vi "Write CAN Frame.vi"(8 "error in (no error)":errorcluster, 10 "data":T1[](array[typedef]) {"payload" format="%x"; "timestamp" format="%<%.7X\n%x>T"; "type" items=["CAN Data"=0, "CAN Remote"=1, "CAN Bus Error"=2, "CAN 2.0 Data"=8, "CAN FD Data"=16, "CAN FD+BRS Data"=24, "J1939 Data"=192, "Delay"=224, "Log Trigger"=225, "Start Trigger"=226]; "identifier" format="%x"}, 11 "PXI 8513 in":refnum<class "PXI 8513.lvclass">) -> (0 "error out":errorcluster, 3 "PXI 8513 out":refnum<class "PXI 8513.lvclass">)   [LabVIEW 2016, in "CAN.lvlib" / "PXI 8513.lvclass"]
uses:
  PXI 8513.lvclass
  <vilib>/xnet/xnet.llb/XNET Frame CAN.ctl
  <vilib>/xnet/xnet.llb/XNET Frame Type CAN.ctl
  PXI 8513.lvclass/PXI 8513.ctl
  <vilib>/xnet/xnet.llb/XNET Write (Frame CAN).vi
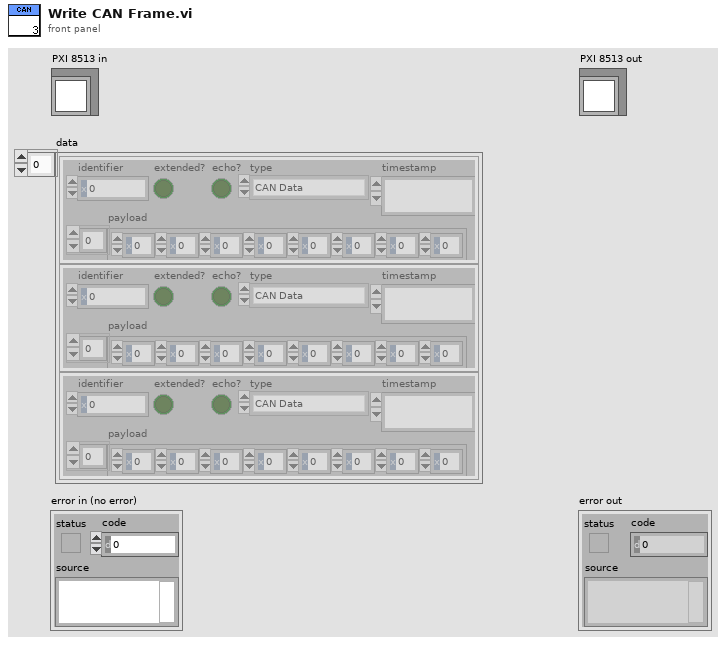
[diagram p1: front panel]
types:
  T1 = typedef "XNET Frame CAN.ctl" = cluster{"timestamp":timestamp, "payload":u8[], "identifier":u32, "type":T2, "extended?":bool, "echo?":bool}
  T2 = typedef "XNET Frame Type CAN.ctl" = u8
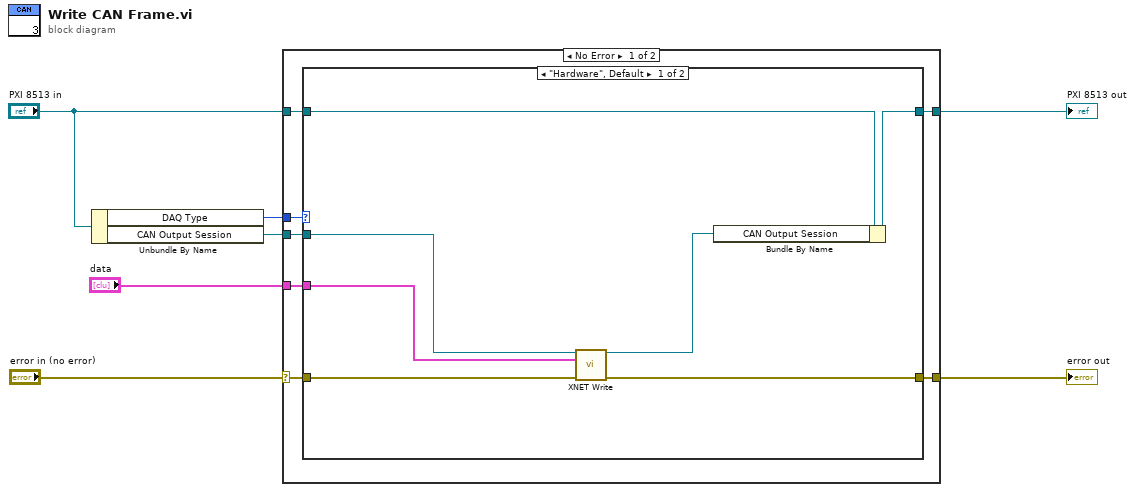
[diagram p0: block diagram]
diagram:
  n1 = Unbundle By Name("PXI 8513 in") -> ("DAQ Type"=w5:enum16{"Hardware", "Simulation"}, "CAN Output Session"=w4:refnum<k21>)
  n2 = case shown="No Error" "error in (no error)" {
    selector: "error in (no error)" -> [w13 w24]
    tunnel: "PXI 8513 in" -> [w10 w25]
    tunnel: w5 -> [w14 _]
    tunnel: w4 -> [w12 _]
    tunnel: "data" -> [w11 _]
    tunnel: [w9 w25] -> w2
    tunnel: [w8 w24] -> w1
    frame No Error {
      n3 = case shown="\"Hardware\", Default" w14 {
        tunnel: w13 -> [w21 w22]
        tunnel: w12 -> [w20 _]
        tunnel: w11 -> [w19 _]
        tunnel: w10 -> [w18 w23]
        tunnel: [w16 w23] -> w9
        tunnel: [w17 w22] -> w8
        frame "Hardware", Default {
          n4 = call-poly <vilib>:"XNET Write.vi"("session in"=w20, "data"=w19, "error in (no error)"=w21) -> ("session out"=w15:refnum<k21>, "error out"=w17:errorcluster)  [unwired: 11 out]
          n5 = Bundle By Name(cluster=w18, "CAN Output Session"=w15) -> (w16:refnum<class "PXI 8513.lvclass">)
        }
        frame "Simulation" {
        }
      }
    }
    frame Error {
    }
  }
  "error out" <- w1
  "PXI 8513 out" <- w2
